vi "rqcBob ServiceNET Send Data Poly.vi"   [LabVIEW 2018]
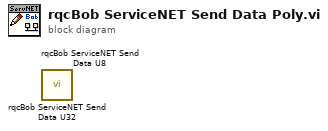
[diagram p0: block diagram]
diagram:
  n1 = call "rqcBob ServiceNET Send Data U32.vi"() -> ()  [unwired: 10 in, 2 out]
  n2 = call "rqcBob ServiceNET Send Data U8.vi"() -> ()  [unwired: 10 in, 2 out]
